vi "Set Elevator Direction off.vi"(8 "error in (no error)":errorcluster, 11 "Elevator Controller in":refnum<class "Elevator Controller.lvclass">) -> (0 "error out":errorcluster, 3 "Elevator Controller out":refnum<class "Elevator Controller.lvclass">)   [LabVIEW 2019, in "Elevator Controller.lvlib" / "Elevator Controller.lvclass"]
uses:
  Elevator Controller.lvclass
  Sim Display Console Actor/Sim Display Console Actor Messages/Write Elevator Direction Msg/Write Elevator Direction Msg.lvclass
  Sim Display Console Actor/Elevator Controller/Elevator Direction.ctl
  Sim Display Console Actor/Elevator Controller/Sim Display Console Actor.lvclass
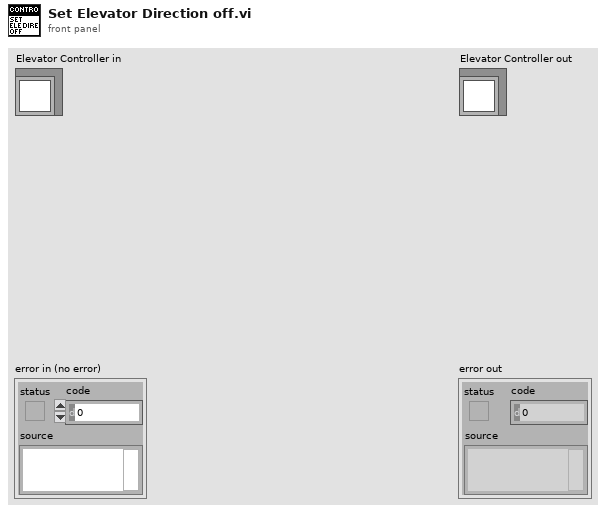
[diagram p1: front panel]
types:
  T1 = typedef "Sim Display Console Actor.lvlib/Sim Display Console Actor.lvclass/Elevator Direction.ctl" = cluster{"Open Door":bool, "Close Door":bool}
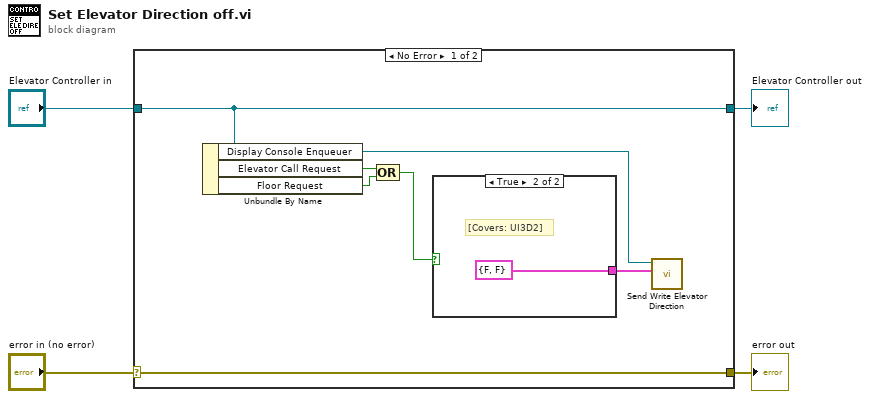
[diagram p0: block diagram]
diagram:
  n1 = case shown="No Error" "error in (no error)" {
    selector: "error in (no error)" -> [w11 w14]
    tunnel: [w11 w14] -> w3
    tunnel: [w10 w13] -> w1
    tunnel: "Elevator Controller in" -> [w10 w13]
    frame No Error {
      n2 = Unbundle By Name(w10) -> ("Display Console Enqueuer"=w7:refnum<class "Message Enqueuer.lvclass">, "Elevator Call Request"=w9:bool, "Floor Request"=w8:bool)
      n3 = Compound Arithmetic op=OR(w9, w8) -> (w5:bool)
      n4 = case shown="True" w5 {
        tunnel: [_ T1 {"Open Door"=FALSE, "Close Door"=FALSE} ("Elevator Direction")] -> w6
        frame False {
        }
        frame True {
          # "[Covers: UI3D2]"
        }
      }
      n5 = call "Send Write Elevator Direction.vi"("Elevator Direction"=w6, "Message Enqueuer"=w7) -> ()  [unwired: 8 in, 2 out]
    }
    frame Error {
    }
  }
  "error out" <- w3
  "Elevator Controller out" <- w1
